vi "Robot Saved.vi"(8 "error in":errorcluster) -> (0 "error out":errorcluster, 2 "RB SAVED?":bool)   [LabVIEW 2016]
uses:
  <vilib>/Rock Robotics/Network Tables/NT Read Boolean.vi
  <vilib>/Rock Robotics/Network Tables/NT Write Boolean.vi
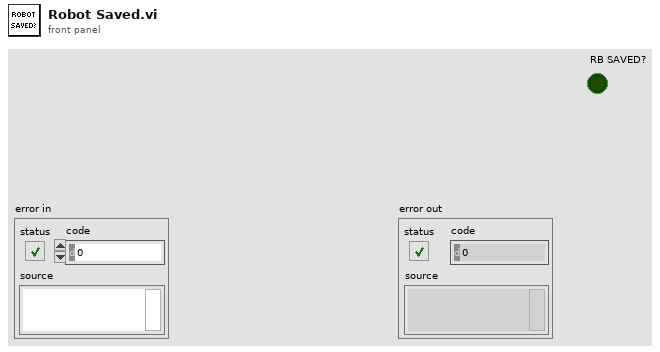
[diagram p1: front panel]
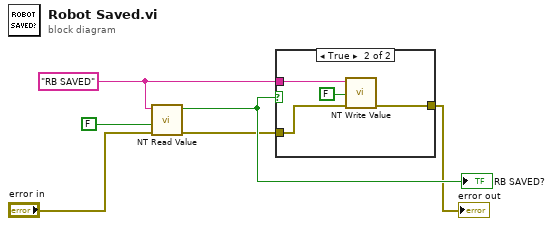
[diagram p0: block diagram]
diagram:
  w3 = "RB SAVED"
  n1 = call-poly <vilib>:"NT Read Value.vi"("error in"="error in", "Default Value"=FALSE, "Name"=w3) -> ("error out"=w2:errorcluster, "Boolean"=w4:bool)  [unwired: 7 in]
  "RB SAVED?" <- w4
  n2 = case shown="True" w4 {
    tunnel: w3 -> [_ w11]
    tunnel: w2 -> [w7 w10]
    tunnel: [w7 w9] -> w1
    frame False {
    }
    frame True {
      n3 = call-poly <vilib>:"NT Write Value.vi"("error in"=w10, "Boolean"=FALSE, "Name"=w11) -> ("error out"=w9:errorcluster)  [unwired: 8 in]
    }
  }
  "error out" <- w1
